vi "Horn_query_junk.vi"(9 "error in (no error)":errorcluster) -> (0 "error out":errorcluster, 2 "connection ID_out":refnum<k5>, 3 "Resonant Frequencies":string)   [LabVIEW 2017]
panel:
  out "*(type *) &x 3":u8
  out "substring":string
  out "data out 2":string
  out "x+y":i32
  out "array":string[](array[string])
  out "*(type *) &x":u8
  # "OUTPUT"
  # "INPUT"
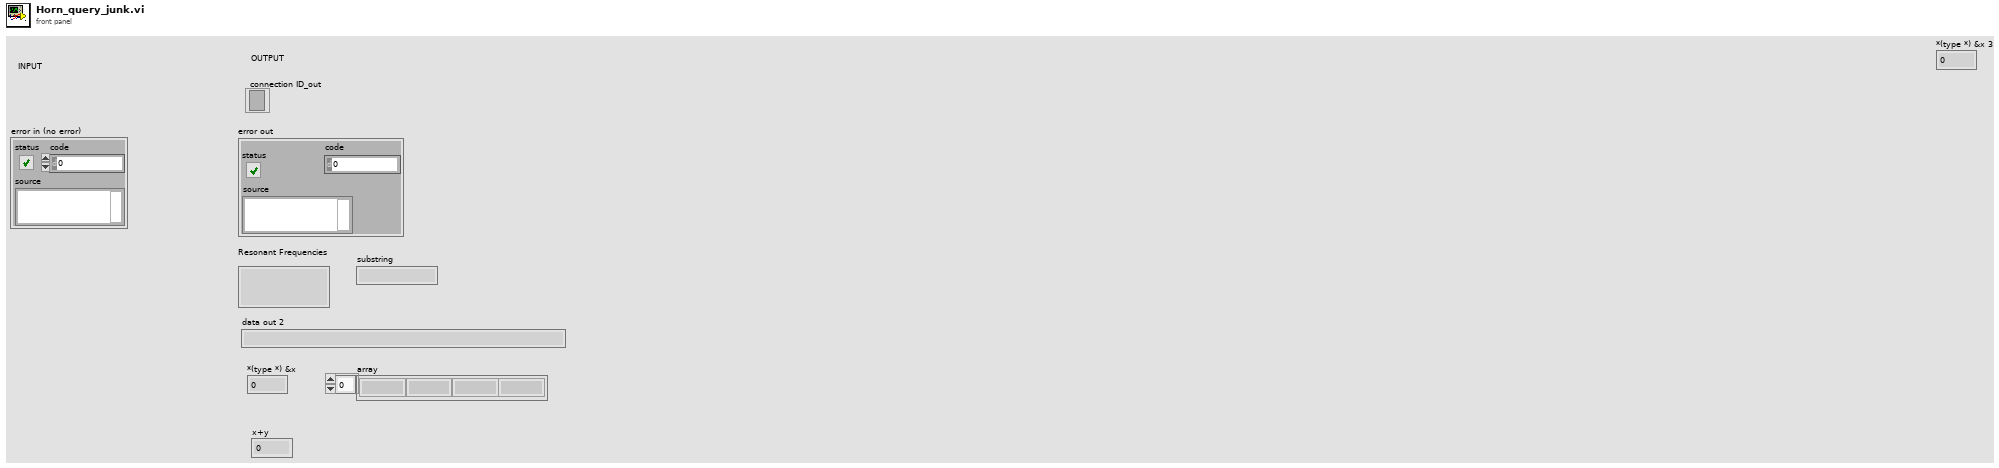
[diagram p1: front panel]
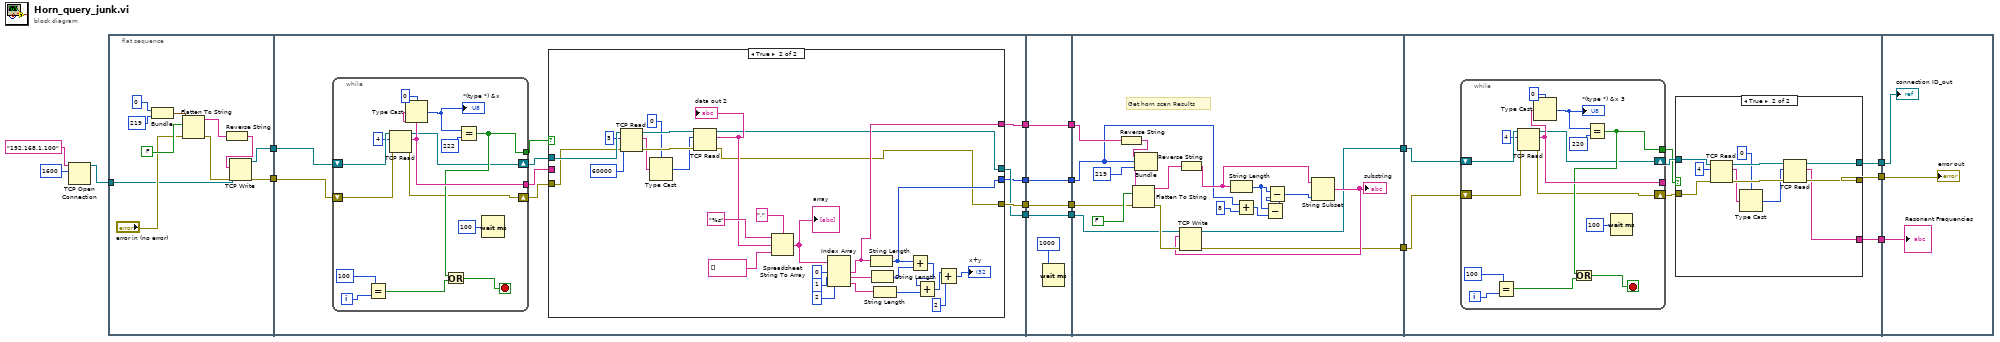
[diagram p0: block diagram]
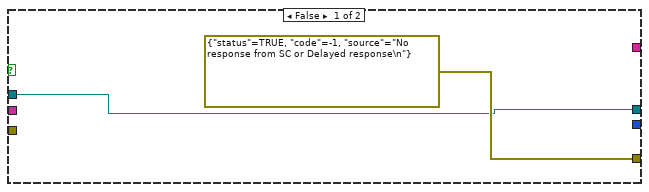
[diagram p2: hidden frame]
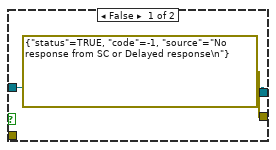
[diagram p3: hidden frame]
diagram:
  n1 = TCP Open Connection(address="192.168.1.100", remote port or service name=u16 1600) -> (connection ID=w3:refnum<k5>)  [unwired: 3 in, 1 out]
  n2 = flat-sequence {
    tunnel: [w25] -> w7
    tunnel: [w24] -> w6
    tunnel: w3 -> [w19]
    tunnel: w7 -> [w37]
    tunnel: w6 -> [w36]
    tunnel: [w34] -> w17
    tunnel: [w32] -> w15
    tunnel: [w31] -> w14
    tunnel: [w30] -> w11
    tunnel: [w89] -> w18
    tunnel: w17 -> [w89]
    tunnel: [w88] -> w16
    tunnel: w15 -> [w88]
    tunnel: w14 -> [w87]
    tunnel: [w87] -> w13
    tunnel: [w86] -> w12
    tunnel: w11 -> [w86]
    tunnel: w18 -> [w106]
    tunnel: w16 -> [w105]
    tunnel: w13 -> [w98]
    tunnel: w12 -> [w103]
    tunnel: [w95] -> w5
    tunnel: [w94] -> w4
    tunnel: w5 -> [w117]
    tunnel: w4 -> [w116]
    tunnel: [w114] -> w10
    tunnel: [w113] -> w9
    tunnel: [w112] -> w8
    tunnel: w10 -> [w147]
    tunnel: w9 -> [w146]
    tunnel: w8 -> [w148]
    frame #0 {
      n3 = Bundle(0, 219) -> (w23:cluster{i32, i32})  [unwired: 1 in]
      n4 = Flatten To String(anything=w23, prepend array or string size? (T)=FALSE, error in (no error)="error in (no error)") -> (data string=w22:string, error out=w28:errorcluster)  [unwired: 1 in, 1 out]
      n5 = Reverse String(1:w22) -> (0:w21:string)
      n6 = TCP Write(connection ID=w19, data in=w21, error in (no error)=w28) -> (connection ID out=w25:refnum<k5>, error out=w24:errorcluster)  [unwired: 1 in, 1 out]
    }
    frame #1 {
      n7 = while {
        shift-right: [w43] -> w33
        shift-left: w37 -> [w45]
        shift-right: [w42] -> w35
        shift-left: w36 -> [w44]
        tunnel: [w47] -> w39
        tunnel: [w51] -> w38
        i -> [w50]
        stop <- w48 stop-if-true
        n8 = Equal?(x=100, y=w50) -> (x = y?=w46:bool)
        n9 = TCP Read(connection ID=w45, bytes to read=4, error in (no error)=w44) -> (connection ID out=w43:refnum<k5>, data out=w51:string, error out=w42:errorcluster)  [unwired: 2 in]
        n10 = Type Cast(type=u8 0, x=w51) -> (*(type *) &x=w53:u8)
        "*(type *) &x" <- w53
        n11 = Equal?(x=w53, y=u8 222) -> (x = y?=w47:bool)
        n12 = Or(x=w47, y=w46) -> (x .or. y?=w48:bool)
        n13 = Wait (ms)(milliseconds to wait=u32 100) -> ()  [unwired: 1 out]
      }
      n14 = case shown="True" w39 {
        tunnel: w38 -> [_ _]
        tunnel: w35 -> [_ w67]
        tunnel: [errorcluster {"status"=TRUE, "code"=-1, "source"="No response from SC or Delayed response\n"} ("error constant") w57] -> w34
        tunnel: w33 -> [w55 w68]
        tunnel: [w55 w58] -> w32
        tunnel: [_ w70] -> w31
        tunnel: [_ w69] -> w30
        frame False {
        }
        frame True {
          n15 = TCP Read(connection ID=w68, bytes to read=5, error in (no error)=w67, 9:60000 ("timeout ms (25000)")) -> (connection ID out=w64:refnum<k5>, data out=w63:string, error out=w65:errorcluster)  [unwired: 1 in]
          n16 = Type Cast(type=u8 0, x=w63) -> (*(type *) &x=w61:u8)
          n17 = TCP Read(connection ID=w64, bytes to read=w61, error in (no error)=w65) -> (connection ID out=w58:refnum<k5>, data out=w60:string, error out=w57:errorcluster)  [unwired: 2 in]
          "data out 2" <- w60
          n18 = Spreadsheet String To Array(delimiter (Tab)=",", format string="%s", spreadsheet string=w60, array type (2D Dbl)=string[] []) -> (array=w82:string[])
          "array" <- w82
          n19 = Index Array(array=w82, index #1=0 ("index"), index #2=1 ("index"), index #3=2 ("index")) -> (element #1=w69:string, element #2=w78:string, element #3=w77:string)
          n20 = String Length(string=w69) -> (length=w70:i32)
          n21 = String Length(string=w78) -> (length=w76:i32)
          n22 = String Length(string=w77) -> (length=w74:i32)
          n23 = Add(x=w70, y=w76) -> (x+y=w75:i32)
          n24 = Add(x=w75, y=w74) -> (x+y=w73:i32)
          n25 = Add(x=w73, y=2) -> (x+y=→"x+y":i32)
        }
      }
    }
    frame #2 {
      n26 = Wait (ms)(milliseconds to wait=u32 1000) -> ()  [unwired: 1 out]
    }
    frame #3 {
      # "Get horn scan Results"
      n27 = Reverse String(1:w103) -> (0:w102:string)
      n28 = Bundle(w102, w98, 219) -> (w101:cluster{string, i32, i32})  [unwired: 1 in]
      n29 = Flatten To String(anything=w101, prepend array or string size? (T)=FALSE, error in (no error)=w106) -> (data string=w107:string, error out=w108:errorcluster)  [unwired: 1 in, 1 out]
      n30 = Reverse String(1:w107) -> (0:w100:string)
      n31 = String Length(string=w100) -> (length=w93:i32)
      n32 = Add(x=w98, y=8 ("bytes to read")) -> (x+y=w92:i32)
      n33 = Subtract(x=w93, y=w92) -> (x-y=w97:i32)
      n34 = Subtract(x=w93, y=w97) -> (x-y=w91:i32)
      n35 = String Subset(string=w100, length (rest)=w91) -> (substring=w96:string)  [unwired: 1 in]
      "substring" <- w96
      n36 = TCP Write(connection ID=w105, data in=w96, error in (no error)=w108) -> (connection ID out=w94:refnum<k5>, error out=w95:errorcluster)  [unwired: 1 in, 1 out]
    }
    frame #4 {
      n37 = while {
        shift-right: [w134] -> w115
        shift-left: w116 -> [w136]
        shift-right: [w133] -> w110
        shift-left: w117 -> [w135]
        tunnel: [w138] -> w111
        tunnel: [w142] -> _
        i -> [w141]
        stop <- w139 stop-if-true
        n38 = Equal?(x=100, y=w141) -> (x = y?=w137:bool)
        n39 = TCP Read(connection ID=w136, bytes to read=4, error in (no error)=w135) -> (connection ID out=w134:refnum<k5>, data out=w142:string, error out=w133:errorcluster)  [unwired: 2 in]
        n40 = Type Cast(type=u8 0, x=w142) -> (*(type *) &x=w144:u8)
        "*(type *) &x 3" <- w144
        n41 = Equal?(x=w144, y=u8 220) -> (x = y?=w138:bool)
        n42 = Or(x=w138, y=w137) -> (x .or. y?=w139:bool)
        n43 = Wait (ms)(milliseconds to wait=u32 100) -> ()  [unwired: 1 out]
      }
      n44 = case shown="True" w111 {
        tunnel: w115 -> [w118 w124]
        tunnel: [w118 w123] -> w114
        tunnel: [errorcluster {"status"=TRUE, "code"=-1, "source"="No response from SC or Delayed response\n"} ("error constant") w122] -> w113
        tunnel: [_ w121] -> w112
        tunnel: w110 -> [_ w120]
        frame False {
        }
        frame True {
          n45 = TCP Read(connection ID=w124, bytes to read=4, error in (no error)=w120) -> (connection ID out=w128:refnum<k5>, data out=w127:string, error out=w129:errorcluster)  [unwired: 2 in]
          n46 = Type Cast(type=u8 0, x=w127) -> (*(type *) &x=w125:u8)
          n47 = TCP Read(connection ID=w128, bytes to read=w125, error in (no error)=w129) -> (connection ID out=w123:refnum<k5>, data out=w121:string, error out=w122:errorcluster)  [unwired: 2 in]
        }
      }
    }
    frame #5 {
      "error out" <- w146
      "Resonant Frequencies" <- w148
      "connection ID_out" <- w147
    }
  }
